vi "Opgave 2.040 B.vi"() -> ()   [LabVIEW 2022 SP3]
panel:
  out "Numeric":dbl
  out "Array":dbl[](array[numeric])
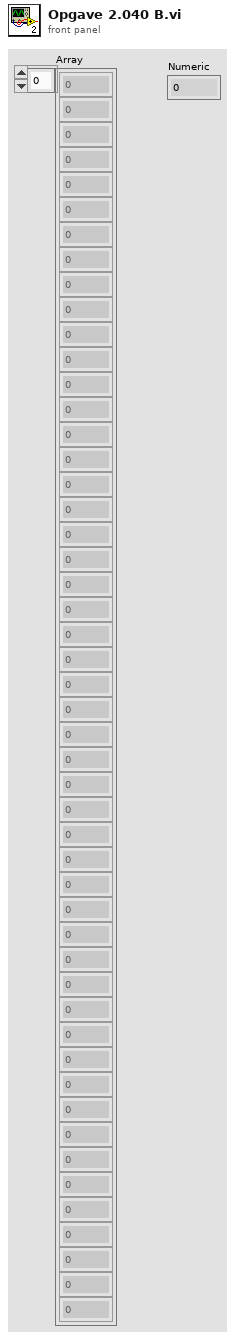
[diagram p1: front panel]
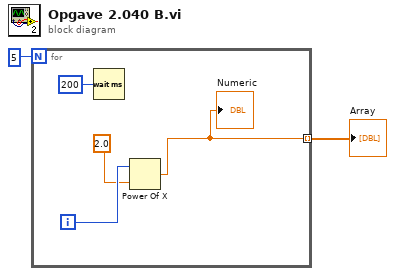
[diagram p0: block diagram]
diagram:
  n1 = for {
    N: 5 -> [_]
    tunnel: [w5] -> w1 mode=indexing
    i -> [w4]
    n2 = Wait (ms)(milliseconds to wait=u32 200) -> ()  [unwired: 1 out]
    n3 = Power Of X(1:2.0 ("y"), 2:w4) -> (0:w5:dbl)
    "Numeric" <- w5
  }
  "Array" <- w1
